vi "Wektor ostatni elem.vi"(11 "wektor":dbl[](array[numeric])) -> (3 "ostatni":dbl)   [LabVIEW 2014]
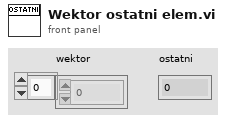
[diagram p1: front panel]
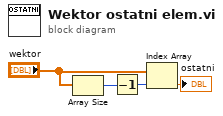
[diagram p0: block diagram]
diagram:
  n1 = Array Size(array="wektor") -> (size(s)=w3:i32)
  n2 = Decrement(x=w3) -> (x-1=w2:i32)
  n3 = Index Array(array="wektor", index=w2) -> (element=→"ostatni":dbl)
